vi "HW CMDs Split.vi"(11 "queryresult":string[][](array[string])) -> (3 "Array":string[][](array[string]))   [LabVIEW 2020]
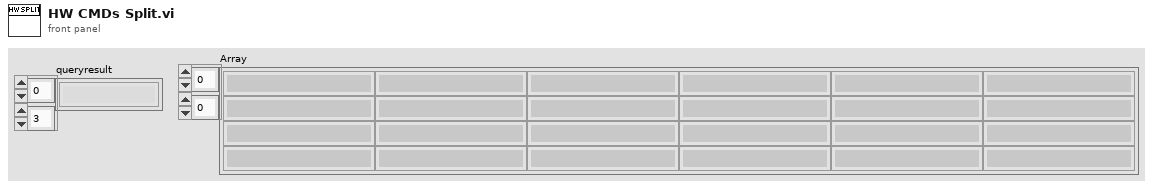
[diagram p1: front panel]
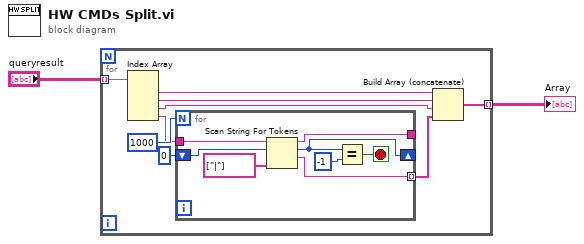
[diagram p0: block diagram]
diagram:
  n1 = for {
    tunnel: "queryresult" -> [w11] mode=indexing
    tunnel: [w8] -> w1 mode=indexing
    n2 = Index Array(array=w11) -> (element #1=w9:string, element #2=w6:string, element #3=w5:string, element #4=w4:string)  [unwired: 4 in]
    n3 = for {
      N: 1000 -> [_]
      tunnel: [w17] -> _
      shift-right: [w13] -> _
      shift-left: 0 ("offset past token") -> [w12]
      tunnel: w4 -> [w18]
      tunnel: [w16] -> w10 mode=indexing
      stop <- w15 stop-if-true
      n4 = Scan String For Tokens(6:string[] ["|"] ("delimiters (\\s,\\t,\\r,\\n)"), 8:w12, 9:w18) -> (1:w16:string, 2:w13:i32, 3:w17:string)  [unwired: 3 in, 1 out]
      n5 = Equal?(x=w13, y=-1) -> (x = y?=w15:bool)
    }
    n6 = Build Array (concatenate)(w9, w6, w5, w10) -> (w8:string[])
  }
  "Array" <- w1
